vi "RT VI.vi"() -> ()   [LabVIEW 2020]
uses:
  <vilib>/rvi/interface/nirviCloseFPGA/nirviCloseFPGA.xnode
  <vilib>/rvi/interface/nirviOpenFPGA/nirviOpenFPGA.xnode
  <vilib>/rvi/interface/nirviReadWriteControl/nirviReadWriteControl.xnode
  <vilib>/rvi/interface/Simulation/niFpgaSimulationCallBeginRW.vi
  <vilib>/rvi/errors/niLvFpgaAdjustHostInterfaceError.vi
  FPGA Bitfiles/rtfpgatestversio_FPGATarget2_fpgaVI_p6Dea0uDK5o.lvbitx
  fpgaVI.vi
  <vilib>/FPGAPlugInAG/Dynamic/niLvFpga_Close_Dynamic.vi
panel:
  out "NI 9263":dbl
  in  "Anode Enable":bool
  in  "ANODE VOLTAGE":dbl(slide) min=0.0 max=10000.0 step=0.183 scale=0.0..10000.0 scale format="%#_7f"
  in  "Kp":dbl
  in  "Ki":dbl
  in  "Kd":dbl
  out "Current Voltage":dbl
  in  "?":bool
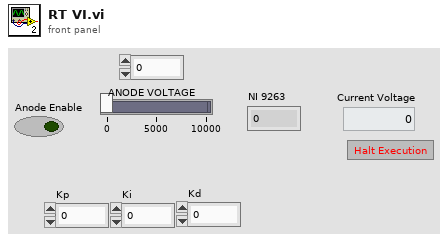
[diagram p1: front panel]
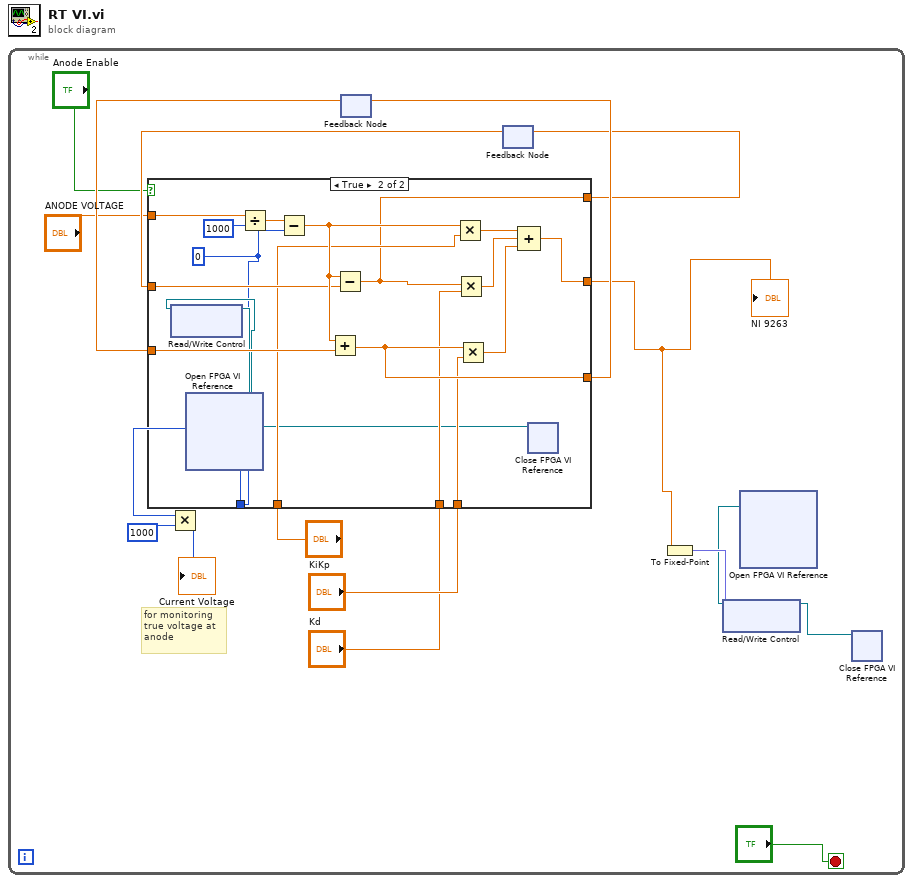
[diagram p0: block diagram]
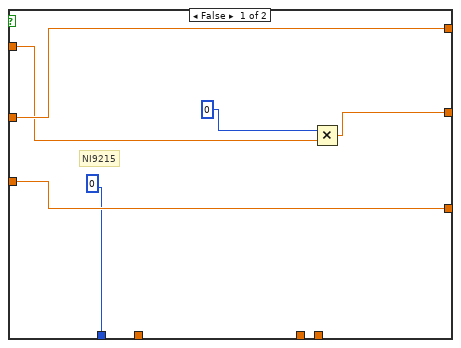
[diagram p2: hidden frame]
diagram:
  n1 = while {
    stop <- "?" stop-if-true
    # "for monitoring \ntrue voltage at\nanode"
    n2 = feedback #1() -> (w16:dbl)  [unwired: 1 in]
    n3 = feedback #2() -> (w17:dbl)  [unwired: 1 in]
    n4 = case shown="True" "Anode Enable" {
      tunnel: w17 -> [w23 w35]
      tunnel: [w23 w25] -> w7
      tunnel: w16 -> [w22 w34]
      tunnel: [w22 w33] -> w12
      tunnel: "ANODE VOLTAGE" -> [w20 w32]
      tunnel: [w19 w31] -> w1
      tunnel: "Kp" -> [_ w30]
      tunnel: "Ki" -> [_ w29]
      tunnel: "Kd" -> [_ w28]
      tunnel: [0 w24] -> w8
      frame False {
        # "NI9215"
        n5 = Multiply(x=0, y=w20) -> (x*y=w19:dbl)
      }
      frame True {
        w24 = 0
        n6 = xnode "Open FPGA VI Reference"() -> ("FPGA VI Reference Out"=w26:refnum<k20>)  [unwired: 2 in, 1 out]
        n7 = xnode "Read/Write Control"("FPGA VI Reference In"=w26) -> ("FPGA VI Reference Out"=w27:refnum<k20>)  [unwired: 1 in, 2 out]
        n8 = Divide(x=w32, y=1000) -> (x/y=w37:dbl)
        n9 = Subtract(x=w37, y=w24) -> (x-y=w40:dbl)
        n10 = Add(x=w40, y=w34) -> (x+y=w33:dbl)
        n11 = Subtract(x=w40, y=w35) -> (x-y=w25:dbl)
        n12 = Multiply(x=w40, y=w30) -> (x*y=w38:dbl)
        n13 = Multiply(x=w25, y=w28) -> (x*y=w36:dbl)
        n14 = Multiply(x=w33, y=w29) -> (x*y=w39:dbl)
        n15 = Compound Arithmetic op=ADD(w38, w36, w39) -> (w31:dbl)
        n16 = xnode "Close FPGA VI Reference"("FPGA VI Reference In"=w27) -> ()  [unwired: 1 in, 1 out]
      }
    }
    "NI 9263" <- w1
    n17 = Multiply(x=w8, y=1000) -> (x*y=→"Current Voltage":i32)
    n18 = feedback-in #1(w12) -> ()
    n19 = feedback-in #2(w7) -> ()
    n20 = To Fixed-Point(number=w1) -> (fixed-point=w5:fxp<+/-,20,5>)  [unwired: 1 in]
    n21 = xnode "Open FPGA VI Reference"() -> ("FPGA VI Reference Out"=w3:refnum<k20>)  [unwired: 2 in, 1 out]
    n22 = xnode "Read/Write Control"("FPGA VI Reference In"=w3, "Mod4/AO0"=w5) -> ("FPGA VI Reference Out"=w4:refnum<k20>)  [unwired: 1 in, 1 out]
    n23 = xnode "Close FPGA VI Reference"("FPGA VI Reference In"=w4) -> ()  [unwired: 1 in, 1 out]
  }
